vi "Six 8-bit Ports Digital Output.vi"(2 "Packet":u64, 4 "Six 8-bit DO Ports":T1={"8-bit DO Port0"="Chassis1/Mod3/DO7:0", "8-bit DO Port1"="Chassis1/Mod3/DO7:0", "8-bit DO Port2"="Chassis1/Mod3/DO7:0", "8-bit DO Port3"="Chassis1/Mod3/DO7:0", "8-bit DO Port4"="Chassis1/Mod3/DO7:0", "8-bit DO Port5"="Chassis1/Mod3/DO7:0"}) -> ()   [LabVIEW 2009]
uses:
  <vilib>/eio/EIONode/EIONode.xnode
  <vilib>/rvi/eio/nirviEIOImplementation/nirviEIOImplementation.xnode
  <vilib>/rvi/eio/common/nirviEmuTemplateMethod_noerrors.vi
  <vilib>/rvi/eio/common/nirviEmuClasses.ctl
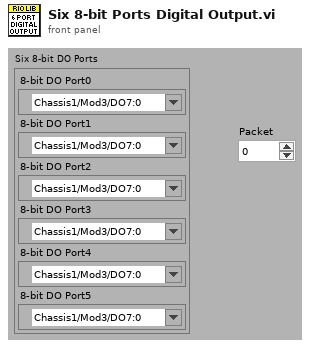
[diagram p1: front panel]
types:
  T1 = cluster{"8-bit DO Port0":refnum<k21>, "8-bit DO Port1":refnum<k21>, "8-bit DO Port2":refnum<k21>, "8-bit DO Port3":refnum<k21>, "8-bit DO Port4":refnum<k21>, "8-bit DO Port5":refnum<k21>}
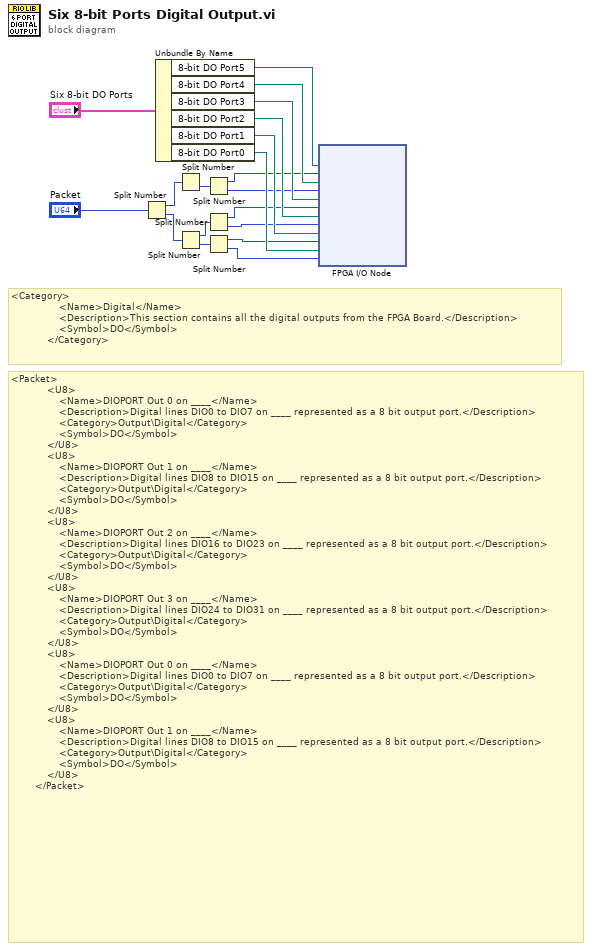
[diagram p0: block diagram]
diagram:
  # "<Packet>\n            <U8>\n                <Name>DIOPORT Out 0 on ____</Name>\n                <Description>Digital lines DIO0 to DIO7 on ____ represented as a 8 bit output port.</Description>\n                <Category>Output\\Digital</Category>\n                <Symbol>DO</Symbol>\n            </U8>\n            <U8>\n                <Name>DIOPORT Out 1 on ____</Name>\n                <Description>Digital lines DIO8 to DIO15 on ____ represented as a 8 bit output port.</Description>\n                <Category>Output\\Digital</Category>\n                <Symbol>DO</Symbol>\n            </U8>\n            <U8>\n                <Name>DIOPORT Out 2 on ____</Name>\n                <Description>Digital lines DIO16 to DIO23 on ____ represented as a 8 bit output port.</Description>\n                <Category>Output\\Digital</Category>\n                <Symbol>DO</Symbol>\n            </U8>\n            <U8>\n                <Name>DIOPORT Out 3 on ____</Name>\n                <Description>Digital lines DIO24 to DIO31 on ____ represented as a 8 bit output port.</Description>\n                <Category>Output\\Digital</Category>\n                <Symbol>DO</Symbol>\n            </U8>\n            <U8>\n                <Name>DIOPORT Out 0 on ____</Name>\n                <Description>Digital lines DIO0 to DIO7 on ____ represented as a 8 bit output port.</Description>\n                <Category>Output\\Digital</Category>\n                <Symbol>DO</Symbol>\n            </U8>\n            <U8>\n                <Name>DIOPORT Out 1 on ____</Name>\n                <Description>Digital lines DIO8 to DIO15 on ____ represented as a 8 bit output port.</Description>\n                <Category>Output\\Digital</Category>\n                <Symbol>DO</Symbol>\n            </U8>\n        </Packet>"
  # "<Category>\n                <Name>Digital</Name>\n                <Description>This section contains all the digital outputs from the FPGA Board.</Description>\n                <Symbol>DO</Symbol>\n            </Category>"
  n1 = Split Number(x="Packet") -> (hi(x)=w5:u32, lo(x)=w18:u32)
  n2 = Unbundle By Name("Six 8-bit DO Ports") -> ("8-bit DO Port5"=w2:refnum<k21>, "8-bit DO Port4"=w6:refnum<k21>, "8-bit DO Port3"=w8:refnum<k21>, "8-bit DO Port2"=w11:refnum<k21>, "8-bit DO Port1"=w14:refnum<k21>, "8-bit DO Port0"=w13:refnum<k21>)
  n3 = Split Number(x=w5) -> (lo(x)=w4:u16)  [unwired: 1 out]
  n4 = Split Number(x=w18) -> (hi(x)=w10:u16, lo(x)=w19:u16)
  n5 = Split Number(x=w4) -> (hi(x)=w1:u8, lo(x)=w3:u8)
  n6 = Split Number(x=w10) -> (hi(x)=w7:u8, lo(x)=w9:u8)
  n7 = Split Number(x=w19) -> (hi(x)=w12:u8, lo(x)=w17:u8)
  n8 = xnode "FPGA I/O Node"("I/O Item"=w1, "I/O Item"=w3, "I/O Item"=w7, "I/O Item"=w9, "I/O Item"=w12, "I/O Item"=w17, "FPGA I/O In"=w2, "FPGA I/O In"=w6, "FPGA I/O In"=w8, "FPGA I/O In"=w11, "FPGA I/O In"=w14, "FPGA I/O In"=w13) -> ()  [unwired: 6 out]
